vi "SUB_appendText_File.vi"(3 "Append Text":string, 4 "Text String on the first line":string, 5 "file_name":string) -> ()   [LabVIEW 2011]
panel:
  out "err code":i32
  out "error out":errorcluster
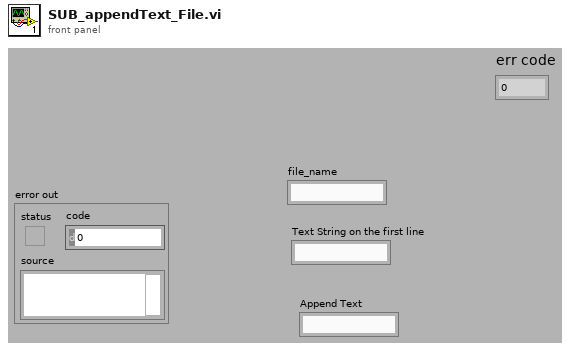
[diagram p1: front panel]
types:
  T1 = enum32{"invalid app kind", "Development System", "Run Time System", "Student Edition", "Embedded LabVIEW", "Evaluation", "Custom"}
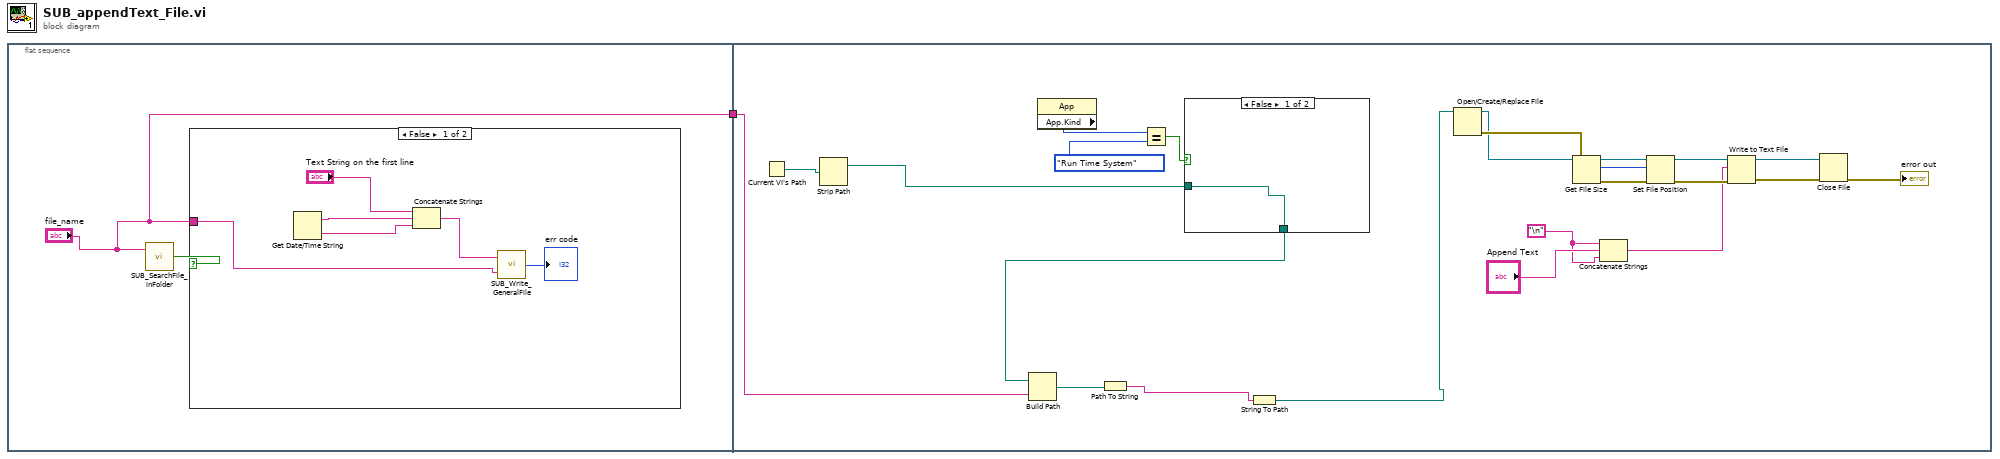
[diagram p0: block diagram]
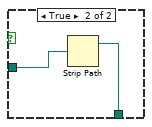
[diagram p3: hidden frame]
diagram:
  n1 = flat-sequence {
    tunnel: ["file_name"] -> w1
    tunnel: w1 -> [w10]
    frame #0 {
      n2 = call "SUB_SearchFile_inFolder.vi"("Search Filename in Folder"="file_name") -> ("File Existing True/Flase"=w3:bool)  [unwired: 1 in]
      n3 = case shown="False" w3 {
        tunnel: "file_name" -> [w5 _]
        frame False {
          n4 = Get Date/Time String() -> (date string=w9:string, time string=w8:string)  [unwired: 3 in]
          n5 = Concatenate Strings("Text String on the first line", w9, w8) -> (w6:string)
          n6 = call "SUB_Write_GeneralFile.vi"("Filename"=w5, "Text Input"=w6) -> ("err code"=→"err code":i32)
        }
        frame True {
        }
      }
    }
    frame #1 {
      w12 = "\n"
      n7 = Current VI's Path() -> (path=w22:path)
      n8 = Strip Path(path=w22) -> (stripped path=w18:path)  [unwired: 1 out]
      n9 = property class="App"() -> ("App.Kind"=w21:T1)  [unwired: 2 in, 2 out]
      n10 = Equal?(x=w21, y=T1."Run Time System" ("Application:Kind")) -> (x = y?=w19:bool)
      n11 = case shown="False" w19 {
        tunnel: w18 -> [w33 w35]
        tunnel: [w33 w34] -> w16
        frame False {
        }
        frame True {
          n12 = Strip Path(path=w35) -> (stripped path=w34:path)  [unwired: 1 out]
        }
      }
      n13 = Build Path(base path=w16, name or relative path=w10) -> (appended path=w17:path)
      n14 = Path To String(path=w17) -> (string=w15:string)
      n15 = String To Path(string=w15) -> (path=w14:path)
      n16 = Open/Create/Replace File(file path (use dialog)=w14) -> (refnum out=w31:refnum<file>, error out=w32:errorcluster)  [unwired: 5 in, 1 out]
      n17 = Get File Size(file=w31, error in=w32) -> (refnum out=w28:refnum<file>, size (in bytes)=w29:i64, 0:w30:errorcluster)
      n18 = Concatenate Strings(w12, "Append Text", w12) -> (w11:string)
      n19 = Set File Position(offset (in bytes) (0)=w29, refnum=w28, error in=w30) -> (refnum out=w27:refnum<file>, error out=w26:errorcluster)  [unwired: 1 in]
      n20 = Write to Text File(file (use dialog)=w27, text=w11, error in=w26) -> (refnum out=w24:refnum<file>, error out=w25:errorcluster)  [unwired: 1 in, 1 out]
      n21 = Close File(refnum=w24, error in=w25) -> (error out=→"error out":errorcluster)  [unwired: 1 out]
    }
  }
